vi "Find SDI Address.vi"(8 "error in (no error)":errorcluster, 11 "H3611i Actor in":refnum<class "H3611i Actor.lvclass">) -> (0 "error out":errorcluster, 3 "H3611i Actor out":refnum<class "H3611i Actor.lvclass">)   [LabVIEW 2018, in "H3611i.lvlib" / "H3611i Actor.lvclass"]
doc: "This VI is meant for use after calling 'Configure H3611i.vi' It scans available SDI addresses, starting with most common, and sets the H3611i object's private data with it's address and parent data with the sensor's serial number."
uses:
  H3611i Actor.lvclass
  C:/Users/dev/Documents/CODE/LabVIEW/microwaveverify/trunk/MWWL Verification/Sensor Actor/Sensor/Sensor.lvclass
  H3611i Actor.lvclass/H3611i Actor.ctl
  Sensor Actor/Sensor/Sensor.lvclass
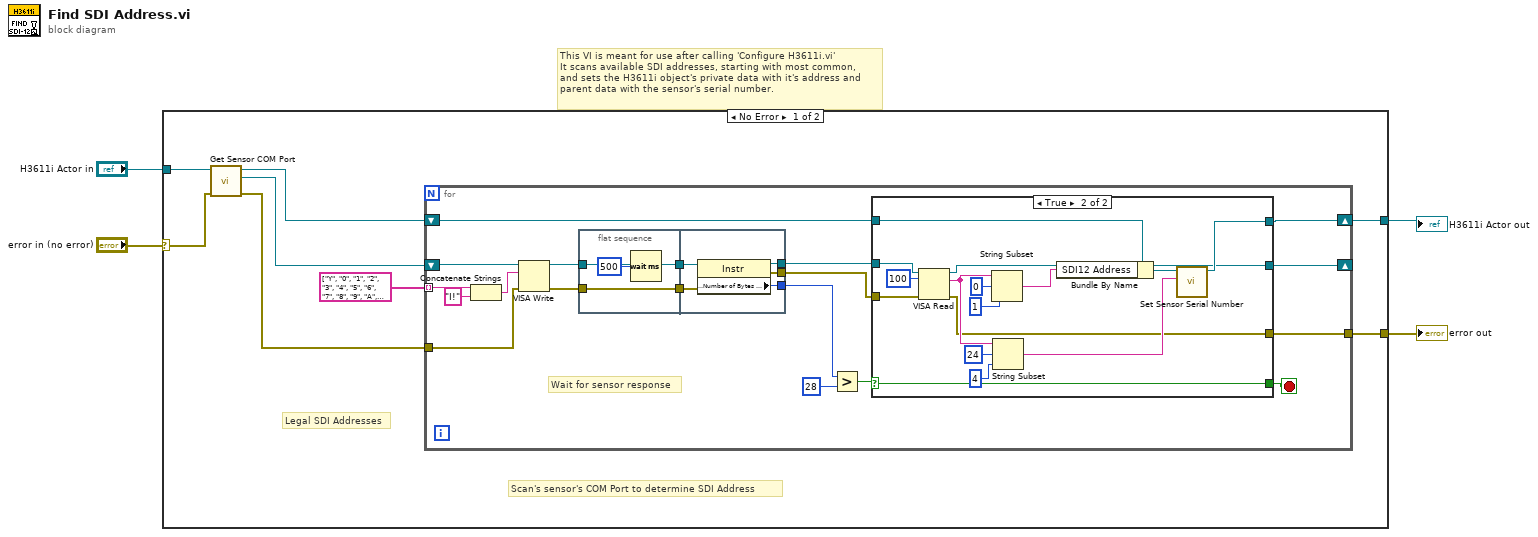
[diagram p0: block diagram]
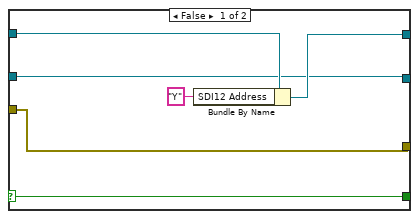
[diagram p2: hidden frame]
diagram:
  # "This VI is meant for use after calling 'Configure H3611i.vi'\nIt scans available SDI addresses, starting with most common,\nand sets the H3611i object's private data with it's address and\nparent data with the sensor's serial number."
  n1 = case shown="No Error" "error in (no error)" {
    selector: "error in (no error)" -> [w11 w63]
    tunnel: [w5 w63] -> w3
    tunnel: [w7 w62] -> w1
    tunnel: "H3611i Actor in" -> [w12 w62]
    frame No Error {
      # "Legal SDI Addresses"
      # "Scan's sensor's COM Port to determine SDI Address"
      n2 = call "Get Sensor COM Port.vi"("error in (no error)"=w11, "Sensor in"=w12) -> ("error out"=w6:errorcluster, "COM Port"=w10:refnum<visa-resource-name>, "Sensor out"=w8:refnum<class "H3611i Actor.lvclass">)  [unwired: 7 in]
      n3 = for {
        tunnel: string[] ["Y", "0", "1", "2", "3", "4", "5", "6", "7", "8", "9", "A", "B", "C", "D", "E", "F", "G", "H", "I", "J", "K", "L", "M", "N", "O", "P", "Q", "R", "S", "T", "U", "V", "W", "X", "Z", "a", "b", "c", "d", "e", "f", "g", "h", "i", "j", "k", "l", "m", "n", "o", "p", "q", "r", "s", "t", "w", "x", "y", "z"] -> [w30] mode=indexing
        shift-right: [w18] -> _
        shift-left: w10 -> [w31]
        tunnel: w6 -> [w26]
        tunnel: [w14] -> w5
        shift-right: [w21] -> w7
        shift-left: w8 -> [w22]
        stop <- w13 stop-if-true
        # "Wait for sensor response"
        n4 = Concatenate Strings(w30, "I!" ("string")) -> (w28:string)
        n5 = VISA Write(VISA resource name=w31, write buffer=w28, error in (no error)=w26) -> (VISA resource name out=w24:refnum<visa-resource-name>, error out=w23:errorcluster)  [unwired: 1 out]
        n6 = flat-sequence {
          tunnel: w23 -> [w55]
          tunnel: w24 -> [w56]
          tunnel: [w56] -> w17
          tunnel: [w55] -> w16
          tunnel: [w61] -> w25
          tunnel: [w58] -> w19
          tunnel: [w57] -> w15
          tunnel: w17 -> [w60]
          tunnel: w16 -> [w59]
          frame #0 {
            n7 = Wait (ms)(milliseconds to wait=u32 500) -> ()  [unwired: 1 out]
          }
          frame #1 {
            n8 = property class="Instr"(reference=w60, error in=w59) -> (reference out=w58:refnum<visa-resource-name>, error out=w57:errorcluster, "Serial Settings:Number of Bytes at Serial Port"=w61:u32)
          }
        }
        n9 = Greater?(x=w25, y=u32 28) -> (0:w20:bool)
        n10 = case shown="True" w20 {
          selector: w20 -> [w32 w38]
          tunnel: w22 -> [w37 w53]
          tunnel: [w36 w48] -> w21
          tunnel: w19 -> [w34 w42]
          tunnel: [w34 w41] -> w18
          tunnel: w15 -> [w33 w40]
          tunnel: [w33 w39] -> w14
          tunnel: [w32 w38] -> w13
          frame False {
            n11 = Bundle By Name(cluster=w37, "SDI12 Address"="Y") -> (w36:refnum<class "H3611i Actor.lvclass">)
          }
          frame True {
            n12 = VISA Read(VISA resource name=w42, byte count=u32 100, error in (no error)=w40) -> (VISA resource name out=w41:refnum<visa-resource-name>, read buffer=w43:string, error out=w39:errorcluster)  [unwired: 1 out]
            n13 = String Subset(string=w43, offset (0)=0, length (rest)=1 ("length (rest)")) -> (substring=w50:string)
            n14 = String Subset(string=w43, offset (0)=24, length (rest)=4 ("length (rest)")) -> (substring=w45:string)
            n15 = Bundle By Name(cluster=w53, "SDI12 Address"=w50) -> (w49:refnum<class "H3611i Actor.lvclass">)
            n16 = call "Set Sensor Serial Number.vi"("Serial Number"=w45, "Sensor in"=w49) -> ("Sensor out"=w48:refnum<class "H3611i Actor.lvclass">)  [unwired: 8 in, 1 out]
          }
        }
      }
    }
    frame Error {
    }
  }
  "error out" <- w3
  "H3611i Actor out" <- w1
